vi "boc_6_dc_channels_voltmetr_measurements.vi"(8 "error in (no error)":errorcluster, 11 "UI_in":T1) -> (0 "error out":errorcluster, 2 "Array":dbl[](array[numeric]), 3 "UI out":T1)   [LabVIEW 2017]
uses:
  ui_buttons.ctl
  types/boc_type.ctl
  ui.ctl
  classes/dc_power_supply/DC_power_supply.lvclass
  classes/report/Report.lvclass
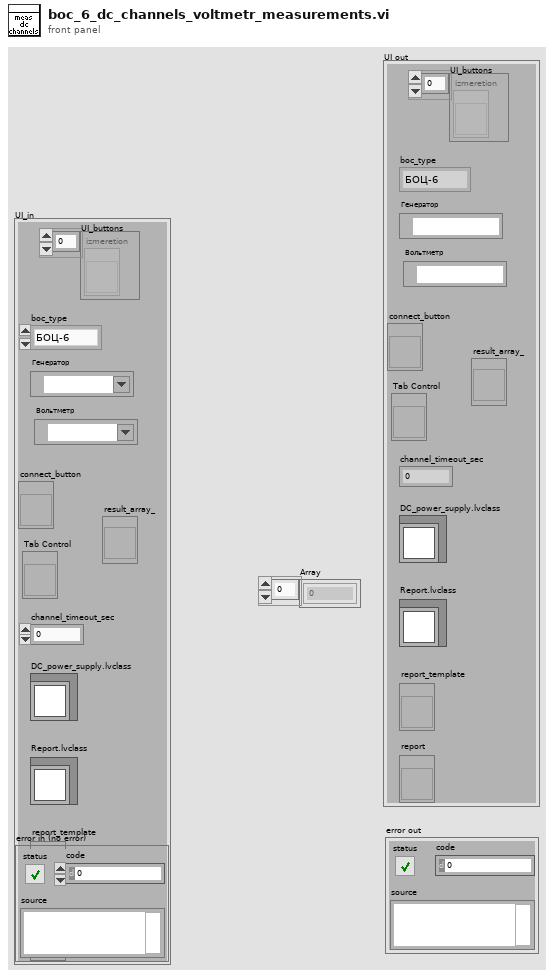
[diagram p1: front panel]
types:
  T1 = typedef "ui.ctl" = cluster{"UI_buttons":T2, "Tab Control":refnum<vi>, "connect_button":refnum<vi>, "generator":refnum<visa-resource-name>, "voltmetr":refnum<visa-resource-name>, "channel_timeout_sec":dbl, "boc_type":T3, "result_array_":refnum<vi>, "DC_power_supply.lvclass":refnum<class "DC_power_supply.lvclass">, "Report.lvclass":refnum<class "Report.lvclass">, "report_template":refnum<vi>, "report":refnum<vi>}
  T2 = typedef "ui_buttons.ctl" = refnum<vi>[]
  T3 = typedef "boc_type.ctl" = enum16{"БОЦ-6", "БОЦ-12"}
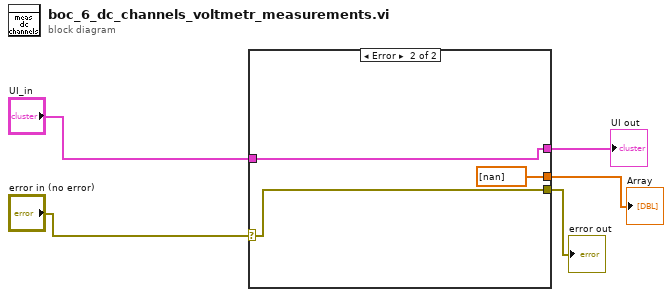
[diagram p0: block diagram]
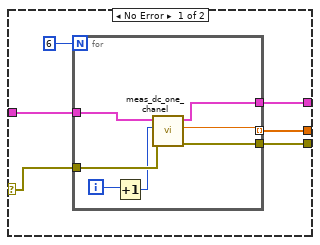
[diagram p2: hidden frame]
diagram:
  n1 = case shown="Error" "error in (no error)" {
    selector: "error in (no error)" -> [w9 w20]
    tunnel: "UI_in" -> [w10 w21]
    tunnel: [w8 w20] -> w3
    tunnel: [w7 w21] -> w2
    tunnel: [w6 dbl[] [nan]] -> w1
    frame No Error {
      n2 = for {
        N: 6 -> [_]
        tunnel: w9 -> [w18]
        tunnel: w10 -> [w17]
        tunnel: [w14] -> w6 mode=indexing
        tunnel: [w13] -> w8
        tunnel: [w12] -> w7
        i -> [w16]
        n3 = Increment(x=w16) -> (x+1=w15:i32)
        n4 = call "meas_dc_one_chanel.vi"("error in (no error)"=w18, "channel"=w15, "UI_out"=w17) -> ("error out"=w13:errorcluster, "Measurement"=w14:dbl, "UI out"=w12:T1)  [unwired: 6 in]
      }
    }
    frame Error {
    }
  }
  "error out" <- w3
  "UI out" <- w2
  "Array" <- w1
